vi "9-libssh2_channel_shell error when pty requested.vi"() -> ()   [LabVIEW 2017, in "bug_reports.lvlib"]
uses:
  bug_reports.lvlib
  libssh2/libssh2_channel_open_ex.vi
  libssh2/libssh2_channel_request_pty_ex.vi
  libssh2/libssh2_channel_process_startup.vi
  support/support.lvlib
  libssh2/libssh2.lvlib
  <vilib>/PNR/Transparent Assertions/Transparent Assertions/Transparent Assertions.lvlib
panel:
  out "error out":errorcluster
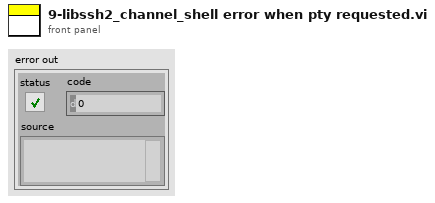
[diagram p1: front panel]
types:
  T1 = typedef "libssh2.lvlib/Session Refnum.ctl" = refnum<k1>
  T2 = typedef "libssh2.lvlib/Channel Refnum.ctl" = refnum<k1>
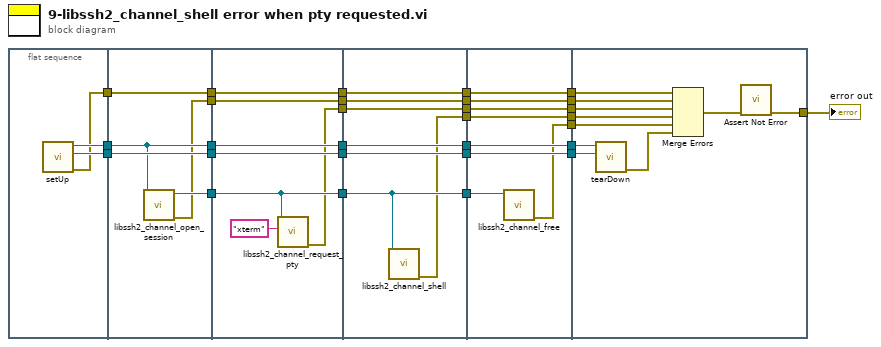
[diagram p0: block diagram]
diagram:
  n1 = flat-sequence {
    tunnel: [w32] -> w29
    tunnel: [w31] -> w28
    tunnel: [w30] -> w27
    tunnel: w29 -> [w36]
    tunnel: w28 -> [w37]
    tunnel: [w36] -> w26
    tunnel: [w37] -> w25
    tunnel: [w35] -> w24
    tunnel: w27 -> [w34]
    tunnel: [w34] -> w23
    tunnel: [w33] -> w22
    tunnel: w26 -> [w44]
    tunnel: w25 -> [w43]
    tunnel: w24 -> [w40]
    tunnel: [w44] -> w15
    tunnel: [w43] -> w13
    tunnel: [w40] -> w11
    tunnel: w23 -> [w42]
    tunnel: [w42] -> w9
    tunnel: w22 -> [w41]
    tunnel: [w41] -> w7
    tunnel: [w38] -> w3
    tunnel: w15 -> [w51]
    tunnel: [w51] -> w14
    tunnel: w13 -> [w50]
    tunnel: [w50] -> w12
    tunnel: w11 -> [w46]
    tunnel: [w46] -> w10
    tunnel: w9 -> [w49]
    tunnel: [w49] -> w8
    tunnel: w7 -> [w48]
    tunnel: [w48] -> w6
    tunnel: [w47] -> w4
    tunnel: w3 -> [w47]
    tunnel: [w45] -> w2
    tunnel: w14 -> [w59]
    tunnel: w12 -> [w58]
    tunnel: w10 -> [w57]
    tunnel: [w59] -> w21
    tunnel: [w58] -> w20
    tunnel: [w56] -> w19
    tunnel: w8 -> [w55]
    tunnel: [w55] -> w18
    tunnel: w6 -> [w54]
    tunnel: [w54] -> w17
    tunnel: [w53] -> w5
    tunnel: w4 -> [w53]
    tunnel: w2 -> [w52]
    tunnel: [w52] -> w1
    tunnel: w21 -> [w69]
    tunnel: w20 -> [w68]
    tunnel: [w67] -> w16
    tunnel: w19 -> [w65]
    tunnel: w18 -> [w64]
    tunnel: w17 -> [w63]
    tunnel: w5 -> [w62]
    tunnel: w1 -> [w60]
    frame #0 {
      n2 = call "setUp.vi"() -> ("error out"=w30:errorcluster, "connection ID"=w31:refnum<k5>, "session"=w32:T1)  [unwired: 9 in]
    }
    frame #1 {
      n3 = call "libssh2_channel_open_session.vi"("session"=w36) -> ("error out"=w33:errorcluster, "channel"=w35:T2)  [unwired: 9 in]
    }
    frame #2 {
      n4 = call "libssh2_channel_request_pty.vi"("term"="xterm", "channel"=w40) -> ("error out"=w38:errorcluster)  [unwired: 9 in]
    }
    frame #3 {
      n5 = call "libssh2_channel_shell.vi"("channel"=w46) -> ("error out"=w45:errorcluster)  [unwired: 10 in]
    }
    frame #4 {
      n6 = call "libssh2_channel_free.vi"("channel"=w57) -> ("error out"=w56:errorcluster)  [unwired: 10 in]
    }
    frame #5 {
      n7 = call "tearDown.vi"("connection ID"=w68, "session"=w69) -> ("error out"=w66:errorcluster)  [unwired: 9 in]
      n8 = Merge Errors(w64, w63, w62, w60, w65, w66) -> (w61:errorcluster)
      n9 = call <vilib>:"Assert Not Error.vi"("error in (no error)"=w61) -> ("error out"=w67:errorcluster)  [unwired: 10 in]
    }
  }
  "error out" <- w16
